vi "Add Node RecursiveChild.vi"(5 "Action":T1, 7 "Delimiter":string, 9 "Node Data":T4, 10 "New Node Path (parent, child)":string[](array[string]), 11 "Tree Map In":T2) -> (0 "error out":errorcluster, 2 "Node Data Replaced?":bool, 3 "Tree Map Out":T2)   [LabVIEW 2020, in "Blue Tree Map OpenSource.lvlib"]
uses:
  Blue Tree Map OpenSource.lvlib
  Typedefs/Tree Node Data.ctl
  Typedefs/Attribute Map.ctl
  Typedefs/Tree Map.ctl
  Typedefs/Tree Map Data.ctl
  Typedefs/AddNodeAction.ctl
  <vilib>/Utility/miscctls.llb/LVMapReplaceAction.ctl
  <vilib>/dlg_ctls.llb/Space Constant.vi
  <vilib>/Utility/error.llb/Error Cluster From Error Code.vi
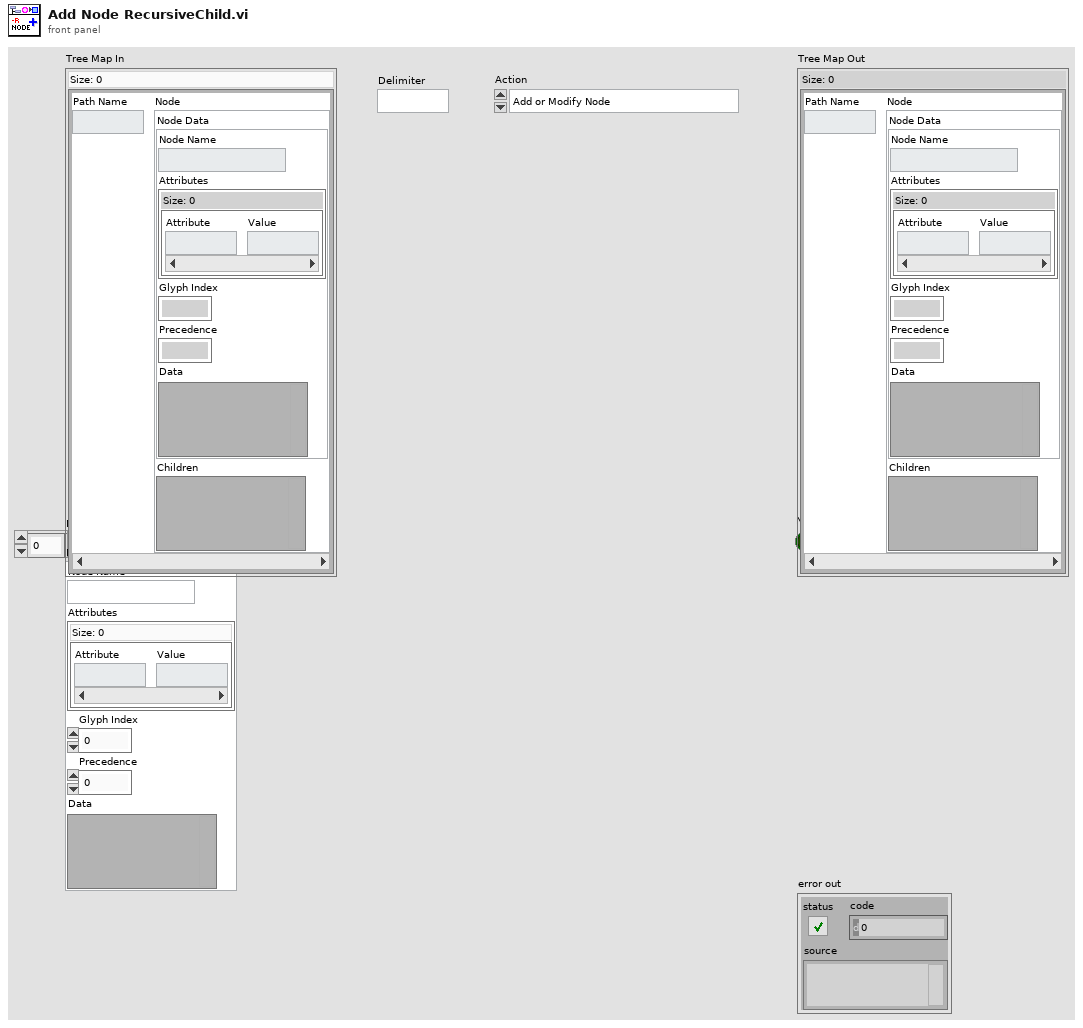
[diagram p1: front panel]
types:
  T1 = typedef "Blue Tree Map OpenSource.lvlib/AddNodeAction.ctl" = enum16{"Add or Modify Node", "Modify Node only if found"}
  T2 = typedef "Blue Tree Map OpenSource.lvlib/Tree Map.ctl" = map{string, T3}
  T3 = typedef "Blue Tree Map OpenSource.lvlib/Tree Map Data.ctl" = cluster{"Node Data":T4, "Children":variant}
  T4 = typedef "Blue Tree Map OpenSource.lvlib/Tree Node Data.ctl" = cluster{"Node Name":string, "Attributes":T5, "Glyph Index":i32, "Precedence":i32, "Data":variant}
  T5 = typedef "Blue Tree Map OpenSource.lvlib/Attribute Map.ctl" = map{string, string}
  T6 = typedef "LVMapReplaceAction.ctl" = enum32{"Modify Entry only if found", "Add or Modify Entry", "Delete Entry"}
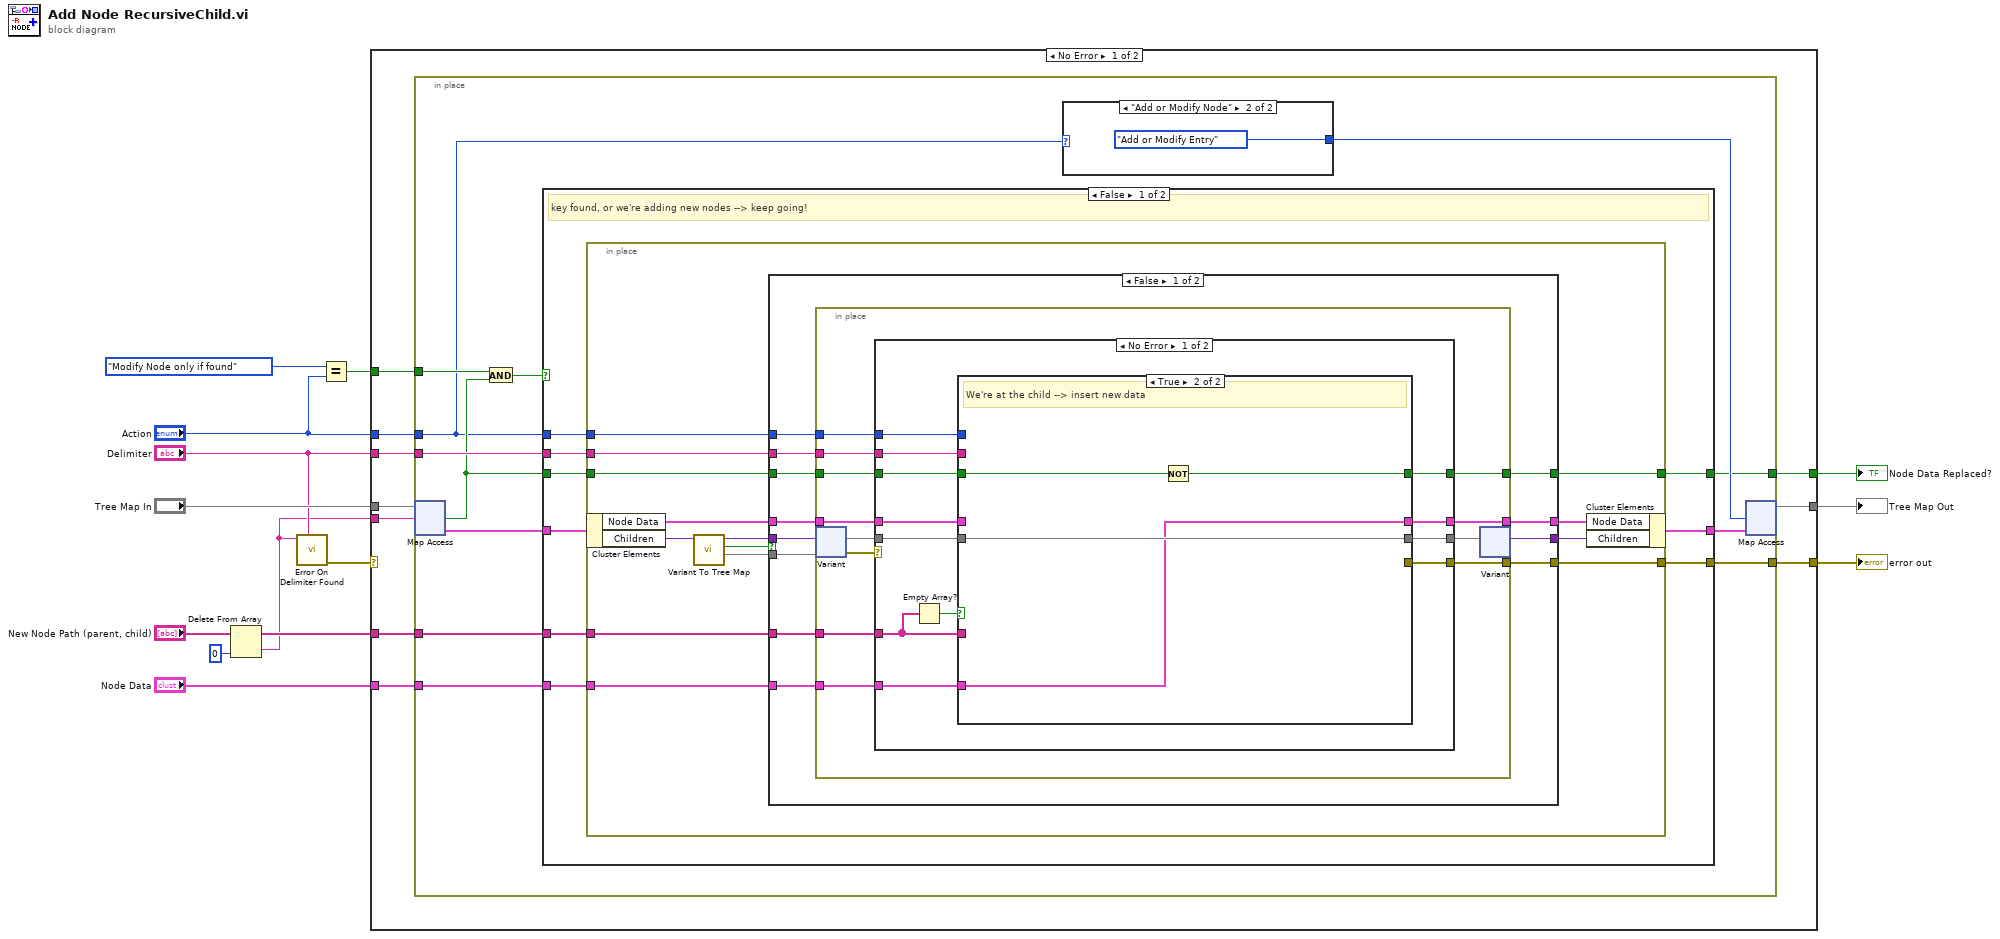
[diagram p0: block diagram]
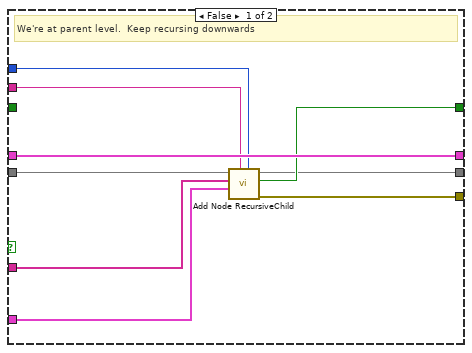
[diagram p2: hidden frame]
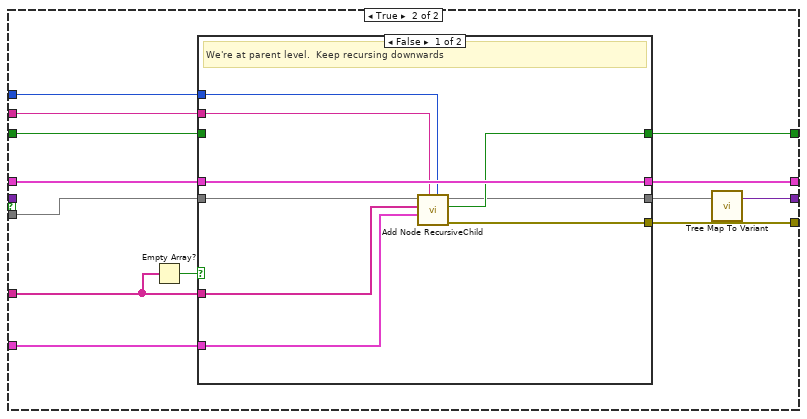
[diagram p4: hidden frame]
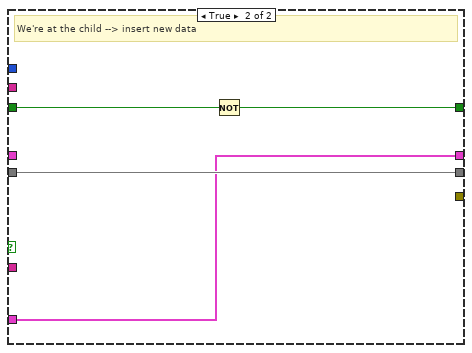
[diagram p5: hidden frame]
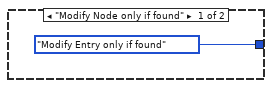
[diagram p7: hidden frame]
diagram:
  n1 = Delete From Array(array="New Node Path (parent, child)", index=0) -> (deleted portion=w1:string, array with subset deleted=w9:string[])  [unwired: 1 in]
  n2 = call "Error On Delimiter Found.vi"("Delimiter"="Delimiter", "Node Path"=w1) -> ("error out"=w8:errorcluster)  [unwired: 9 in]
  n3 = Equal?(x=AddNodeAction."Modify Node only if found" ("Action (Add)"), y="Action") -> (x = y?=w3:bool)
  n4 = case shown="No Error" w8 {
    selector: w8 -> [_ w142]
    tunnel: [w24 w142] -> w13
    tunnel: [w23 _] -> w12
    tunnel: "Node Data" -> [w22 _]
    tunnel: w9 -> [w21 _]
    tunnel: w1 -> [w20 _]
    tunnel: "Tree Map In" -> [w19 w141]
    tunnel: [w18 w141] -> w6
    tunnel: "Delimiter" -> [w17 _]
    tunnel: w3 -> [w16 _]
    tunnel: "Action" -> [w15 _]
    frame No Error {
      n5 = in-place {
        in-place-border: w21 -> [w35]
        in-place-border: w22 -> [w34]
        in-place-border: [w33] -> w24
        in-place-border: [w27] -> w23
        in-place-border: w17 -> [w31]
        in-place-border: w16 -> [w30]
        in-place-border: w15 -> [w25]
        n6 = in-place-map #1(w19, w20) -> (w36:T3, w26:bool)  [unwired: 1 in]
        n7 = And(x=w30, y=w26) -> (x .and. y?=w29:bool)
        n8 = case shown="False" w29 {
          tunnel: w36 -> [w45 w138]
          tunnel: w35 -> [w44 _]
          tunnel: w34 -> [w43 _]
          tunnel: [w42 _] -> w33
          tunnel: [w41 w138] -> w32
          tunnel: w31 -> [w40 _]
          tunnel: [w39 _] -> w27
          tunnel: w26 -> [w38 _]
          tunnel: w25 -> [w37 _]
          frame False {
            # "key found, or we're adding new nodes --> keep going!"
            n9 = in-place {
              in-place-border: w44 -> [w59]
              in-place-border: w43 -> [w58]
              in-place-border: [w56] -> w42
              in-place-border: w40 -> [w54]
              in-place-border: [w53] -> w39
              in-place-border: w38 -> [w52]
              in-place-border: w37 -> [w51]
              n10 = in-place-cluster #2(w45) -> ("Node Data"=w57:T4, "Children"=w49:variant)
              n11 = call "Variant To Tree Map.vi"("Children"=w49) -> ("Tree Map (Empty)"=w47:T2, "Empty?"=w46:bool, "Children"=w48:variant)  [unwired: 8 in]
              n12 = case shown="False" w46 {
                tunnel: w59 -> [w71 w124]
                tunnel: w58 -> [w70 w123]
                tunnel: w57 -> [w69 w122]
                tunnel: [w68 w121] -> w56
                tunnel: [w67 w120] -> w55
                tunnel: w54 -> [w66 w119]
                tunnel: [w65 w118] -> w53
                tunnel: w52 -> [w64 w117]
                tunnel: w51 -> [w63 w116]
                tunnel: [w62 w112] -> w50
                tunnel: w48 -> [w61 _]
                tunnel: w47 -> [w60 w114]
                frame False {
                  n13 = in-place {
                    in-place-border: w71 -> [w73]
                    in-place-border: w70 -> [w83]
                    in-place-border: w69 -> [w82]
                    in-place-border: [w81] -> w68
                    in-place-border: [w80] -> w67
                    in-place-border: w66 -> [w79]
                    in-place-border: [w78] -> w65
                    in-place-border: w64 -> [w77]
                    in-place-border: w63 -> [w76]
                    n14 = in-place-variant #3(w61, w60) -> (w75:T2, w72:errorcluster)
                    n15 = case shown="No Error" w72 {
                      selector: w72 -> [_ w111]
                      tunnel: w83 -> [w95 _]
                      tunnel: w82 -> [w94 w109]
                      tunnel: [w93 w111] -> w81
                      tunnel: [w92 w109] -> w80
                      tunnel: w79 -> [w91 _]
                      tunnel: [w90 _] -> w78
                      tunnel: w77 -> [w89 _]
                      tunnel: w76 -> [w88 _]
                      tunnel: w75 -> [w87 w110]
                      tunnel: [w86 w110] -> w74
                      tunnel: w73 -> [w85 _]
                      frame No Error {
                        n16 = Empty Array?(array=w85) -> (empty?=w84:bool)
                        n17 = case shown="True" w84 {
                          tunnel: w87 -> [w96 w108]
                          tunnel: [w97 w108] -> w86
                          tunnel: w85 -> [w104 _]
                          tunnel: w95 -> [w101 w107]
                          tunnel: [w103 w107] -> w92
                          tunnel: w94 -> [w103 _]
                          tunnel: [w102 _] -> w93
                          tunnel: w91 -> [w100 _]
                          tunnel: [w99 w106] -> w90
                          tunnel: w89 -> [_ w105]
                          tunnel: w88 -> [w98 _]
                          frame False {
                            # "We're at parent level.  Keep recursing downwards"
                            n18 = call "Add Node RecursiveChild.vi"("Action"=w98, "Delimiter"=w100, "Node Data"=w101, "New Node Path (parent, child)"=w104, "Tree Map In"=w96) -> ("error out"=w102:errorcluster, "Node Data Replaced?"=w99:bool, "Tree Map Out"=w97:T2)  [unwired: 4 in]
                          }
                          frame True {
                            # "We're at the child --> insert new data"
                            n19 = Not(x=w105) -> (.not. x?=w106:bool)
                          }
                        }
                      }
                      frame Error {
                      }
                    }
                    n20 = in-place-variant #3(w74) -> (w62:variant)  [unwired: 1 out]
                  }
                }
                frame True {
                  n21 = Empty Array?(array=w124) -> (empty?=w115:bool)
                  n22 = case shown="False" w115 {
                    tunnel: w114 -> [w125 w137]
                    tunnel: [w126 w137] -> w113
                    tunnel: w124 -> [w133 _]
                    tunnel: w123 -> [w130 w136]
                    tunnel: [w132 w136] -> w120
                    tunnel: w122 -> [w132 _]
                    tunnel: [w131 _] -> w121
                    tunnel: w119 -> [w129 _]
                    tunnel: [w128 w135] -> w118
                    tunnel: w117 -> [_ w134]
                    tunnel: w116 -> [w127 _]
                    frame False {
                      # "We're at parent level.  Keep recursing downwards"
                      n23 = call "Add Node RecursiveChild.vi"("Action"=w127, "Delimiter"=w129, "Node Data"=w130, "New Node Path (parent, child)"=w133, "Tree Map In"=w125) -> ("error out"=w131:errorcluster, "Node Data Replaced?"=w128:bool, "Tree Map Out"=w126:T2)  [unwired: 4 in]
                    }
                    frame True {
                      # "We're at the child --> insert new data"
                      n24 = Not(x=w134) -> (.not. x?=w135:bool)
                    }
                  }
                  n25 = call "Tree Map To Variant.vi"("Tree Map"=w113) -> ("Variant"=w112:variant)  [unwired: 2 in]
                }
              }
              n26 = in-place-cluster #2("Node Data"=w55, "Children"=w50) -> (w41:T3)
            }
          }
          frame True {
            # "key not found and we're only modifying nodes --> stop here"
          }
        }
        n27 = case shown="\"Add or Modify Node\"" w25 {
          tunnel: [LVMapReplaceAction."Modify Entry only if found" ("action") LVMapReplaceAction."Add or Modify Entry" ("action")] -> w28
          frame "Modify Node only if found" {
          }
          frame "Add or Modify Node" {
          }
        }
        n28 = in-place-map #1(w32, w28) -> (w18:T2)  [unwired: 2 out]
      }
    }
    frame Error {
    }
  }
  "error out" <- w13
  "Node Data Replaced?" <- w12
  "Tree Map Out" <- w6
